vi "Read turret Angle.vi"(10 "Sensor Gear Ratio":dbl=8.333333333 format="%#_13g", 11 "Input cluster":T1) -> (1 "Turret Angle":dbl(knob) scale=0.0..360.0, 2 "Cumulative Angle":dbl(knob) scale=0.0..360.0)   [LabVIEW 2019]
uses:
  Implementation/Turrent Controller Typedef.ctl
  <vilib>/Rock Robotics/WPI/MotorControl/WPI_MotorControlDeviceRef.ctl
  <vilib>/Rock Robotics/WPI/MotorControl/WPI_MotorControlType.ctl
  <vilib>/Rock Robotics/SystemInterfaces/DIO/FPGA_DIOPWMChannel.ctl
  <vilib>/Rock Robotics/WPI/PWM/WPI_PWMDeadband.ctl
  <vilib>/Rock Robotics/SystemInterfaces/DIO/FPGA_DIOChannel.ctl
  <vilib>/Rock Robotics/SystemInterfaces/DutyCycle/FPGA_DutyCycleDevRef.ctl
  <vilib>/Rock Robotics/SystemInterfaces/DutyCycle/FPGA_DutyCycleIndex.ctl
  <vilib>/Rock Robotics/WPI/Counter/WPI_CounterDevRef.ctl
  <vilib>/Rock Robotics/SystemInterfaces/Counter/FPGA_CounterCtrSystemIndex.ctl
panel:
  out "Absolute Angle":dbl
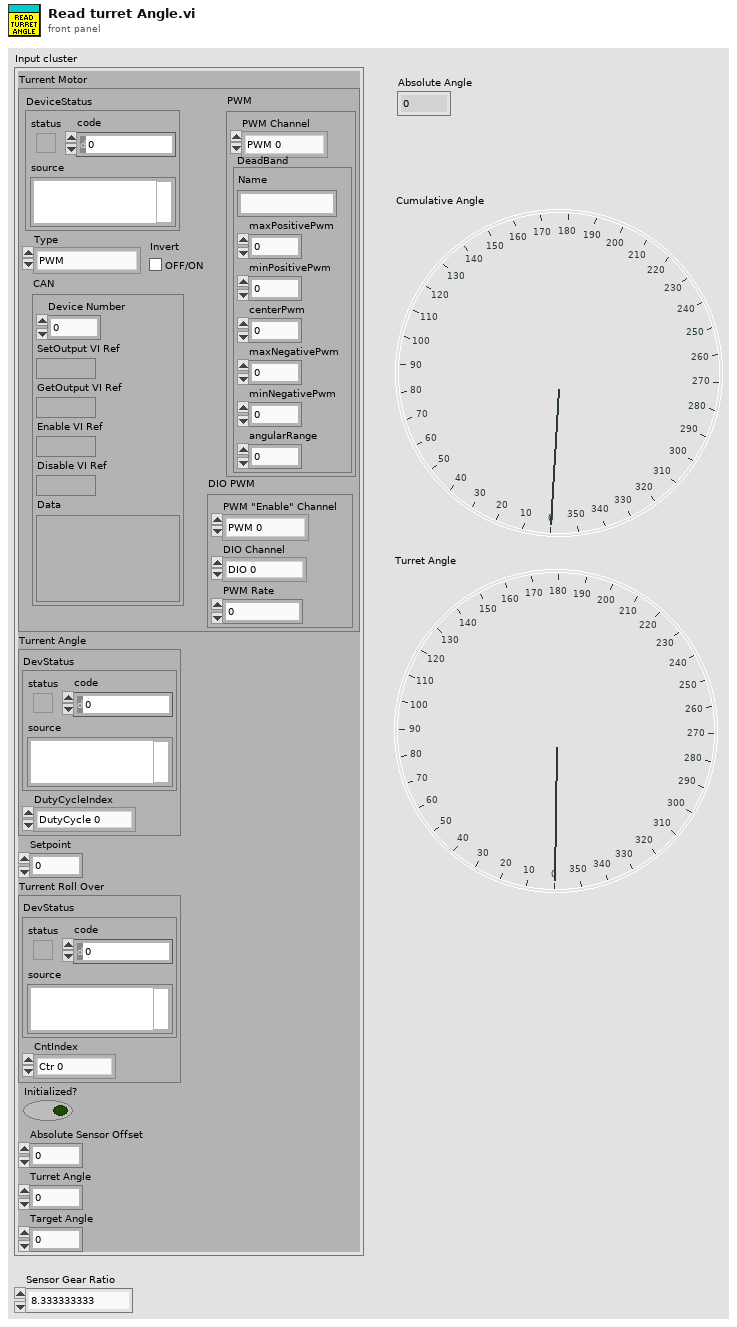
[diagram p1: front panel]
types:
  T1 = typedef "Turrent Controller Typedef.ctl" = cluster{"Turrent Motor":T2, "Turrent Angle":T7, "Setpoint":dbl, "Turrent Roll Over":T9, "Initialized?":bool, "Absolute Sensor Offset":dbl, "Turret Angle":dbl, "Target Angle":dbl}
  T2 = typedef "WPI_MotorControlDeviceRef.ctl" = cluster{"DeviceStatus":errorcluster, "Type":T3, "PWM":cluster{"PWM Channel":T4, "DeadBand":T5}, "CAN":cluster{"Device Number":u8, "SetOutput VI Ref":variant, "GetOutput VI Ref":variant, "Enable VI Ref":variant, "Disable VI Ref":variant, "Data":variant}, "Invert":bool, "DIO PWM":cluster{"PWM \"Enable\" Channel":T4, "DIOChannel":T6, "PWM Rate":dbl}}
  T3 = typedef "WPI_MotorControlType.ctl" = enum16{"PWM", "CAN", "DIO PWM"}
  T4 = typedef "FPGA_DIOPWMChannel.ctl" = enum8{"PWM 0", "PWM 1", "PWM 2", "PWM 3", "PWM 4", "PWM 5", "PWM 6", "PWM 7", "PWM 8", "PWM 9", "PWM MXP 0", "PWM MXP 1", "PWM MXP 2", "PWM MXP 3", "PWM MXP 4", "PWM MXP 5", "PWM MXP 6", "PWM MXP 7", "PWM MXP 8", "PWM MXP 9", "Invalid"}
  T5 = typedef "WPI_PWMDeadband.ctl" = cluster{"Name":string, "maxPositivePwm":i32, "minPositivePwm":i32, "centerPwm":i32, "maxNegativePwm":i32, "minNegativePwm":i32, "angularRange":u16}
  T6 = typedef "FPGA_DIOChannel.ctl" = enum8{"DIO 0", "DIO 1", "DIO 2", "DIO 3", "DIO 4", "DIO 5", "DIO 6", "DIO 7", "DIO 8", "DIO 9", "DIO MXP 0", "DIO MXP 1", "DIO MXP 2", "DIO MXP 3", "DIO MXP 4", "DIO MXP 5", "DIO MXP 6", "DIO MXP 7", "DIO MXP 8", "DIO MXP 9", "DIO MXP 10", "DIO MXP 11", "DIO MXP 12", "DIO MXP 13", "DIO MXP 14", "DIO MXP 15", "SPI Port CS1", "SPI Port CS2", "SPI Port CS3", "SPI Port MISO", "SPI Port MOSI", "Invalid"}
  T7 = typedef "FPGA_DutyCycleDevRef.ctl" = cluster{"DevStatus":errorcluster, "DutyCycleIndex":T8}
  T8 = typedef "FPGA_DutyCycleIndex.ctl" = enum8{"DutyCycle 0", "DutyCycle 1", "DutyCycle 2", "DutyCycle 3", "DutyCycle 4", "DutyCycle 5", "DutyCycle 6", "DutyCycle 7", "Invalid"}
  T9 = typedef "WPI_CounterDevRef.ctl" = cluster{"DevStatus":errorcluster, "CntIndex":T10}
  T10 = typedef "FPGA_CounterCtrSystemIndex.ctl" = enum8{"Ctr 0", "Ctr 1", "Ctr 2", "Ctr 3", "Ctr 4", "Ctr 5", "Ctr 6", "Ctr 7", "Invalid"}
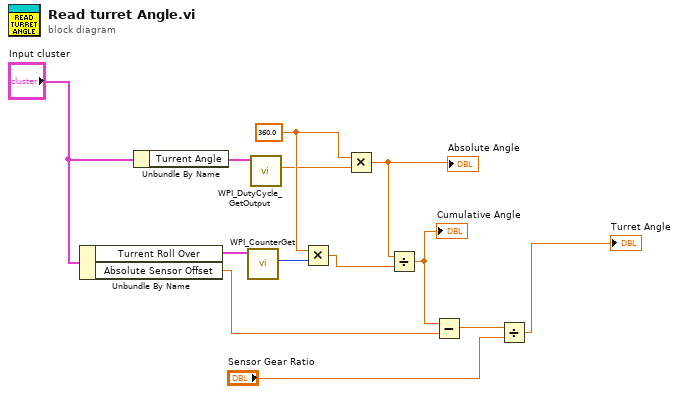
[diagram p0: block diagram]
diagram:
  w4 = 360.0
  n1 = Unbundle By Name("Input cluster") -> ("Turrent Roll Over"=w1:T9, "Absolute Sensor Offset"=w12:dbl)
  n2 = Unbundle By Name("Input cluster") -> ("Turrent Angle"=w5:T7)
  n3 = call <vilib>:"WPI_CounterGet.vi"("CounterDevRef in"=w1) -> ("Value"=w2:i32)  [unwired: 5 in, 5 out]
  n4 = call <vilib>:"WPI_DutyCycle_GetOutput.vi"("DutyCycleDevRef"=w5) -> ("Output"=w3:dbl)  [unwired: 8 in, 2 out]
  n5 = Multiply(x=w4, y=w2) -> (x*y=w7:dbl)
  n6 = Multiply(x=w4, y=w3) -> (x*y=w6:dbl)
  "Absolute Angle" <- w6
  n7 = Divide(x=w6, y=w7) -> (x/y=w8:dbl)
  "Cumulative Angle" <- w8
  n8 = Subtract(x=w8, y=w12) -> (x-y=w9:dbl)
  n9 = Divide(x=w9, y="Sensor Gear Ratio") -> (x/y=→"Turret Angle":dbl)
